vi "Calculate phase.vi"(6 "dV (V)":sgl=0.4 min=0.1 max=5 step=0.1 format="%.1f", 8 "error in (no error)":errorcluster, 10 "Mean values":sgl[](array[numeric]), 11 "Voltages":sgl[](array[numeric])) -> (0 "error out":errorcluster, 2 "Ciclos 2Pi 2":cluster{"xi used":dbl[], "yi":dbl[]}[](graph)=[{"xi used"=[0.0, 0.4000000059604645, 0.800000011920929, 1.2000000476837158, 1.600000023841858, 2.0, 2.4000000953674316, 2.799999952316284, 3.200000047683716, 3.6000001430511475, 4.0, 4.400000095367432, 4.800000190734863, 5.200000286102295, 5.599999904632568, 6.0, 6.400000095367432, 6.800000190734863, 7.200000286102295], "yi"=[1.6194082498550415, 2.081223726272583, 3.9639101028442383, 5.417988300323486, 5.994996547698975, 5.763517379760742, 4.927460193634033, 3.268064022064209, 1.9228070974349976, 2.006049633026123, 3.322584629058838, 5.178757190704346, 5.874281883239746, 5.9817633628845215, 5.3586106300354, 3.7743194103240967, 2.4187028408050537, 2.3153183460235596, 3.7917206287384033]}, {"xi used"=[0.0, 0.10000000149011612, 0.20000000298023224, 0.30000000447034836, 0.4000000059604645, 0.5000000074505806, 0.6000000089406967, 0.7000000104308128, 0.800000011920929, 0.9000000208616257, 1.0000000298023224, 1.100000038743019, 1.2000000476837158, 1.3000000417232513, 1.4000000357627869, 1.5000000298023224, 1.600000023841858, 1.7000000178813934, 1.800000011920929, 1.9000000059604645, 2.0, 2.100000023841858, 2.200000047683716, 2.3000000715255737, 2.4000000953674316, 2.5000000596046448, 2.600000023841858, 2.699999988079071, 2.799999952316284, 2.899999976158142, 3.0, 3.100000023841858, 3.200000047683716, 3.3000000715255737, 3.4000000953674316, 3.5000001192092896, 3.6000001430511475, 3.7000001072883606, 3.8000000715255737, 3.900000035762787, 4.0, 4.100000023841858, 4.200000047683716, 4.300000071525574, 4.400000095367432, 4.5000001192092896, 4.6000001430511475, 4.700000166893005, 4.800000190734863, 4.900000214576721, 5.000000238418579, 5.100000262260437, 5.200000286102295, 5.300000190734863, 5.400000095367432, 5.5, 5.599999904632568, 5.699999928474426, 5.799999952316284, 5.899999976158142, 6.0, 6.100000023841858, 6.200000047683716, 6.300000071525574, 6.400000095367432, 6.5000001192092896, 6.6000001430511475, 6.700000166893005, 6.800000190734863, 6.900000214576721, 7.000000238418579, 7.100000262260437, 7.200000286102295], "yi"=[1.6194082498550415, 1.6415202646400873, 1.700969021152869, 1.835091261121122, 2.081223726272583, 2.4615675244221595, 2.9377812277334487, 3.4563877744572187, 3.9639101028442383, 4.416314498578613, 4.807340439884618, 5.1401707620402455, 5.417988300323486, 5.643229129866736, 5.815342479071086, 5.9330308007455095, 5.994996547698975, 6.0015645873541725, 5.959549445588673, 5.8773880628937665, 5.763517379760742, 5.622745854472534, 5.4453682711596425, 5.218050945615625, 4.927460193634033, 4.566549653810085, 4.153420905030226, 3.7124627576598135, 3.268064022064209, 2.8442846434260165, 2.4638706226251452, 2.1492390703865025, 1.9228070974349976, 1.8016579460584699, 1.7815393847964844, 1.8528653137515367, 2.006049633026123, 2.2327082258196134, 2.529265762805696, 2.8933489839101707, 3.322584629058838, 3.807336769827714, 4.308917005977046, 4.78137419407865, 5.178757190704346, 5.467236063197128, 5.661465721984701, 5.788222288265946, 5.874281883239746, 5.940712665430707, 5.985750942666336, 6.001925060099863, 5.9817633628845215, 5.9173299887642, 5.798831744986865, 5.616011126946077, 5.3586106300354, 5.0225638976458455, 4.628571701943094, 4.203526165358669, 3.7743194103240967, 3.3657338746848104, 2.994113257941885, 2.673691575010305, 2.4187028408050537, 2.2430304554985607, 2.1591553602930404, 2.1792078816481535, 2.3153183460235596, 2.5722541809073114, 2.925331217901028, 3.3425023896347215, 3.7917206287384033]}, {"xi used"=[1.6635191881348852, 5.094512955533968], "yi"=[6.004797437208987, 6.001979760925586]}], 3 "V 2Pi\nActual 2":sgl=3.4309938 format="%#.1g")   [LabVIEW 2020]
uses:
  <vilib>/gmath/NI_Gmath.lvlib
  <vilib>/Analysis/NI_AAL_SigProc.lvlib
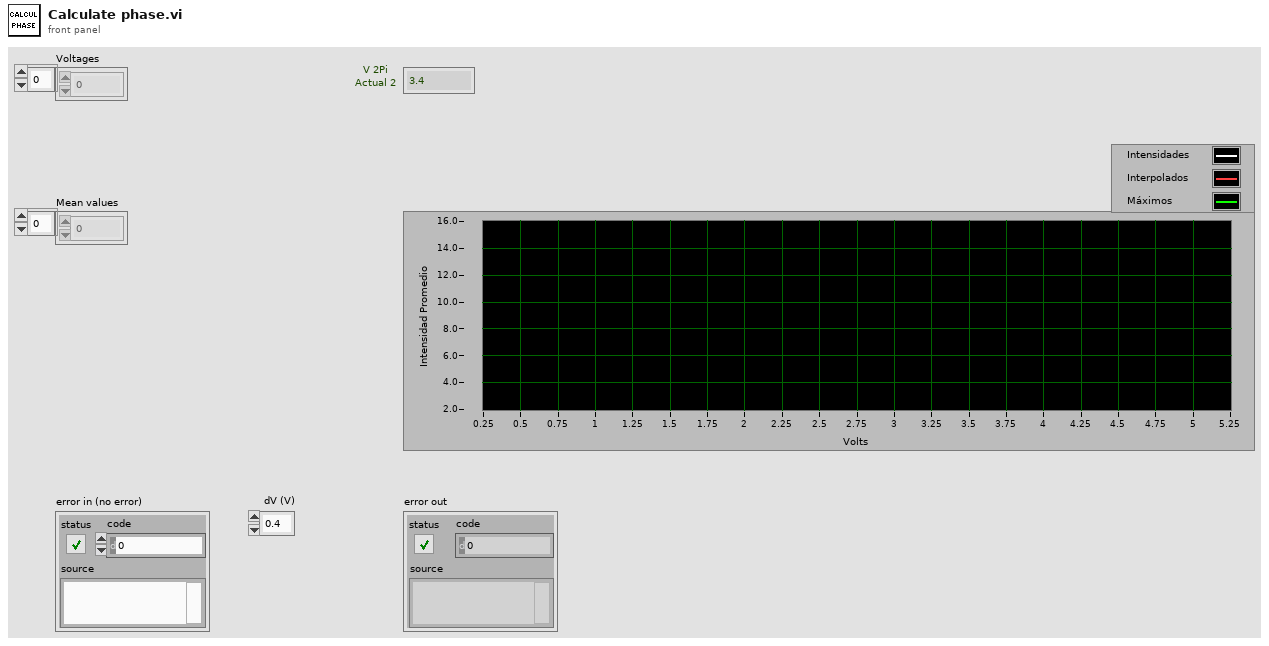
[diagram p1: front panel]
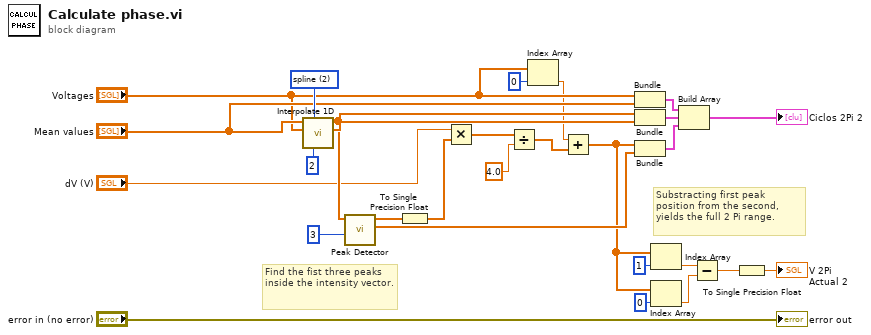
[diagram p0: block diagram]
diagram:
  w24 = 2 items=["nearest", "linear", "spline", "cubic Hermite", "Lagrange"] ("method")
  # "Substracting first peak position from the second, yields the full 2 Pi range."
  # "Find the fist three peaks inside the intensity vector."
  n1 = call <vilib>:"Interpolate 1D.vi"("ntimes"=2, "method"=w24, "X"="Voltages", "Y"="Mean values") -> ("xi used"=w18:dbl[], "yi"=w12:dbl[])  [unwired: 5 in, 1 out]
  n2 = call <vilib>:"Peak Detector.vi"("width"=3, "X"=w12) -> ("Amplitudes"=w10:dbl[], "Locations"=w11:dbl[])  [unwired: 5 in, 3 out]
  n3 = To Single Precision Float(number=w11) -> (single precision float=w1:sgl[])
  n4 = Multiply(x="dV (V)", y=w1) -> (x*y=w17:sgl[])
  n5 = Divide(x=w17, y=sgl 4.0 ("x")) -> (x/y=w16:sgl[])
  n6 = Index Array(array="Voltages", index=0) -> (element=w2:sgl)
  n7 = Add(x=w2, y=w16) -> (x+y=w5:sgl[])
  n8 = Bundle("Voltages"="Voltages", "Mean values"="Mean values") -> (w22:cluster{"Voltages":sgl[], "Mean values":sgl[]})  [unwired: 1 in]
  n9 = Bundle("xi used"=w18, "yi"=w12) -> (w21:cluster{"xi used":dbl[], "yi":dbl[]})  [unwired: 1 in]
  n10 = Bundle(w5, "Amplitudes"=w10) -> (w19:cluster{sgl[], "Amplitudes":dbl[]})  [unwired: 1 in]
  n11 = Index Array(array=w5, index=1) -> (element=w15:sgl)
  n12 = Index Array(array=w5, index=0) -> (element=w14:sgl)
  n13 = Build Array(w22, w21, w19) -> (→"Ciclos 2Pi 2":cluster{"xi used":dbl[], "Amplitudes":dbl[]}[])
  n14 = Subtract(x=w15, y=w14) -> (x-y=w13:sgl)
  n15 = To Single Precision Float(number=w13) -> (single precision float=→"V 2Pi\nActual 2":sgl)
  "error out" <- "error in (no error)"
